vi "ARRAY TUGAS.vi"() -> ()   [LabVIEW 2017]
panel:
  out "Array":i32[](array[numeric])
  in  "Numeric":i32=30
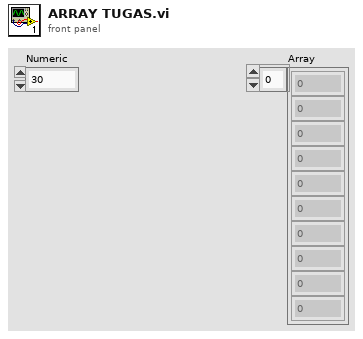
[diagram p1: front panel]
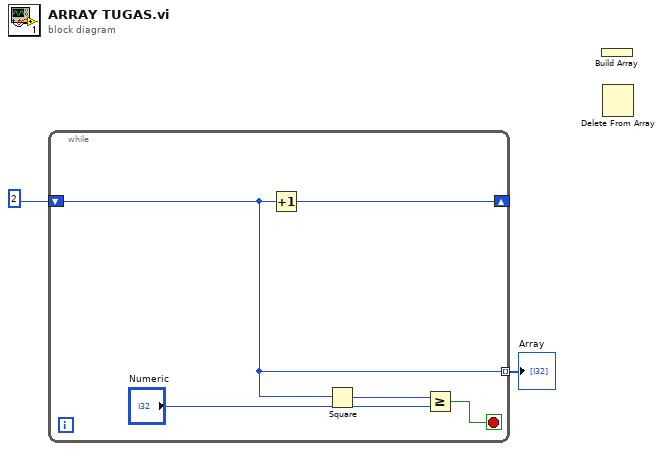
[diagram p0: block diagram]
diagram:
  n1 = while {
    shift-right: [w5] -> _
    shift-left: 2 -> [w3]
    tunnel: [w3] -> w1 mode=indexing
    stop <- w7 stop-if-true
    n2 = Increment(x=w3) -> (x+1=w5:i32)
    n3 = Square(x=w3) -> (x^2=w4:i32)
    n4 = Greater Or Equal?(x=w4, y="Numeric") -> (x >= y?=w7:bool)
  }
  "Array" <- w1
  n5 = Build Array() -> ()  [unwired: 1 in, 1 out]
  n6 = Delete From Array() -> ()  [unwired: 3 in, 2 out]
